vi "TDC读取_32b.vi"() -> ()   [LabVIEW 2014]
uses:
  <vilib>/Utility/file.llb/Write To Spreadsheet File (I64).vi
panel:
  in  "设定测量时间/秒":dbl
  out "测量进行时间/秒":dbl
  out "初始时间":u32
  in  "存储文件路径":path=path "C:/Users/Lebron/Desktop/tdc测试数据/Plain3/10ns.txt" caption="文件路径 （空时为对话框）"
  in  "停止":bool
  out "时间分布谱":dbl[](graph)
  in  "基路径":path=path "C:/Users/Lebron/Desktop/zxd/数据"
  out "路径":path
  in  "下拉列表":u16(ring) items=["继续", "停止"]
  out "状态":enum16{"空闲", "开始", "接收数据", "处理数据", "退出"}(ring)
  out "开关":bool
  in  "通道电压阈值":u16=500
  in  "开始":bool
  in  "初始状态":enum16{"空闲", "开始", "接收数据", "处理数据", "退出"}(ring)
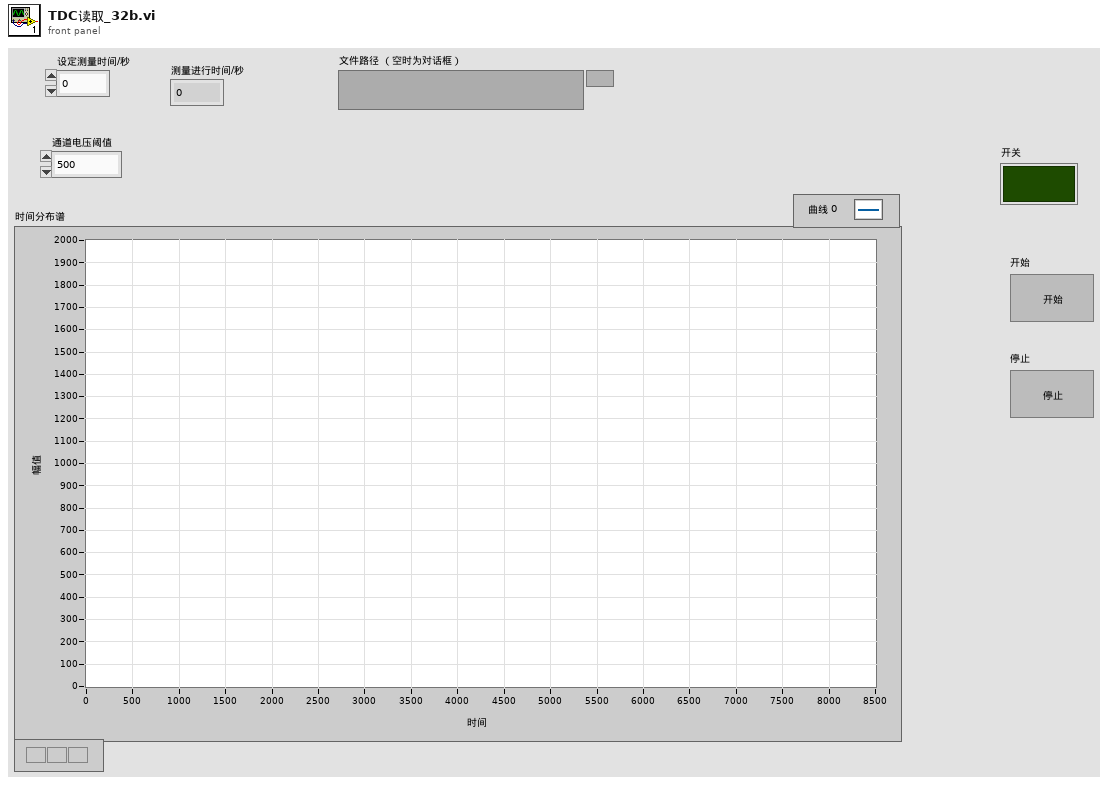
[diagram p1: front panel]
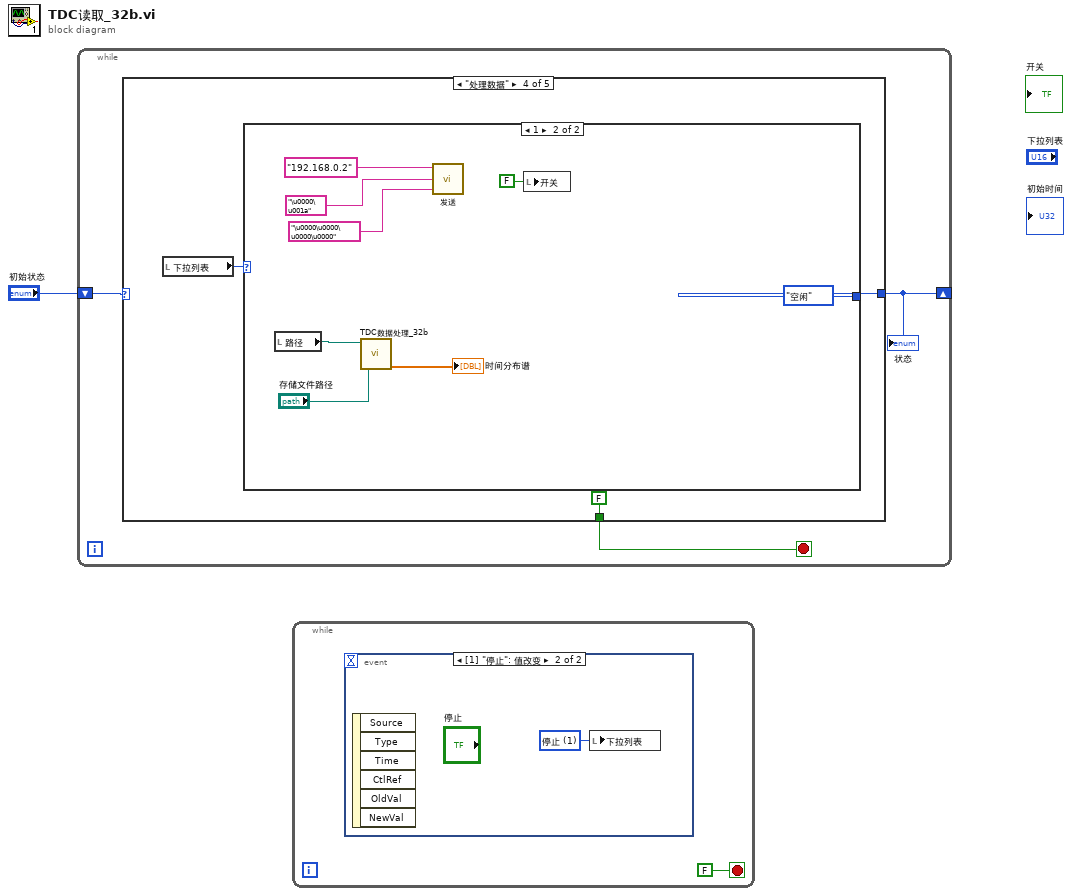
[diagram p0: block diagram]
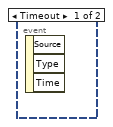
[diagram p2: hidden frame]
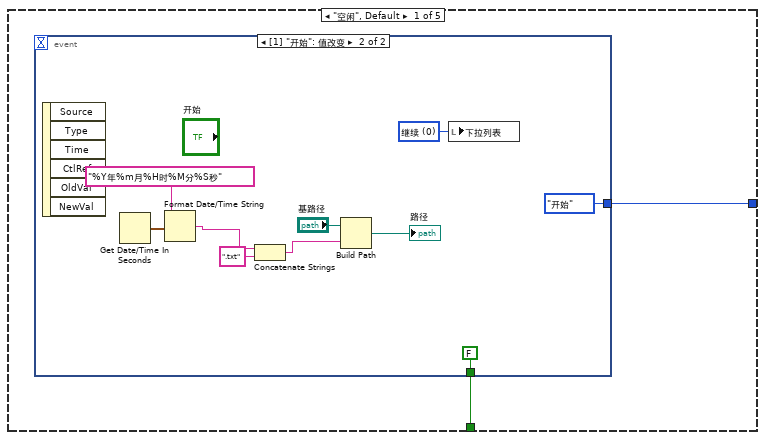
[diagram p3: hidden frame]
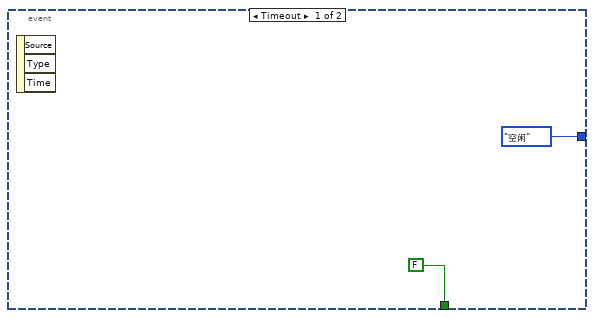
[diagram p4: hidden frame]
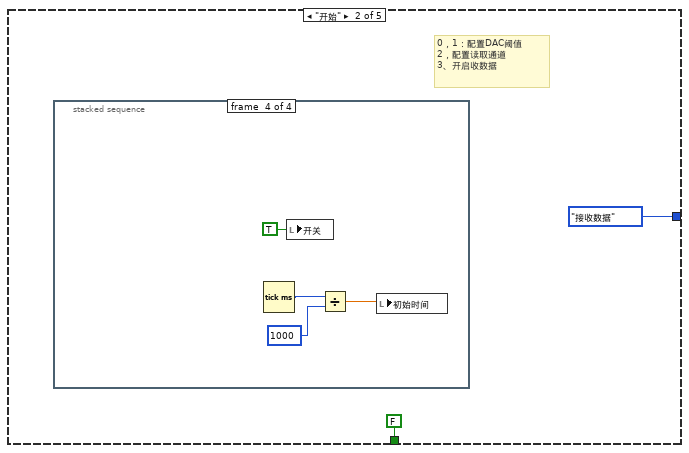
[diagram p5: hidden frame]
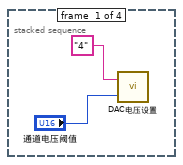
[diagram p6: hidden frame]
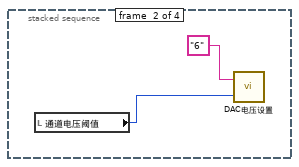
[diagram p7: hidden frame]
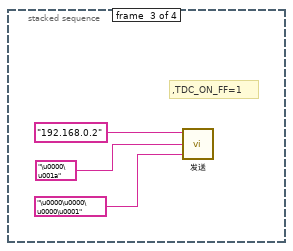
[diagram p8: hidden frame]
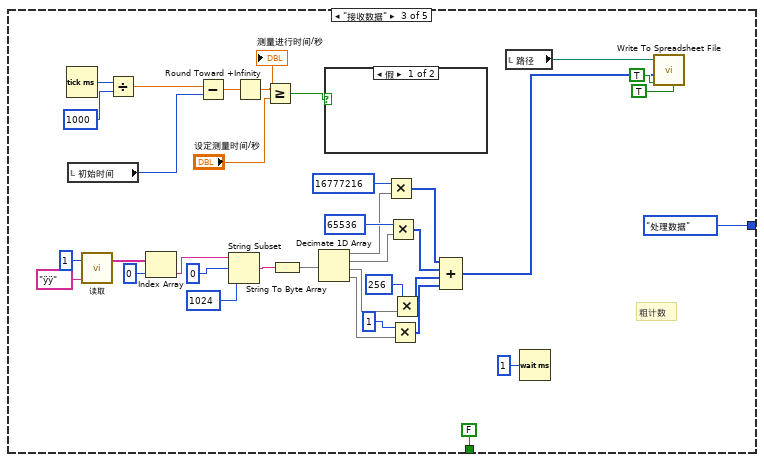
[diagram p9: hidden frame]
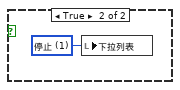
[diagram p10: hidden frame]
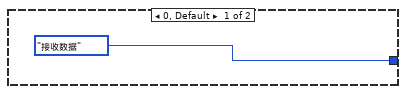
[diagram p11: hidden frame]
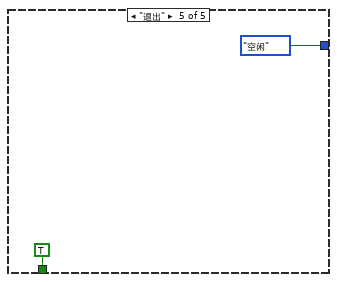
[diagram p12: hidden frame]
diagram:
  n1 = while {
    shift-right: [w3] -> _
    shift-left: "初始状态" -> [w4]
    stop <- w2 stop-if-true
    n2 = case shown="\"处理数据\"" w4 {
      tunnel: [w6 enum16{"空闲", "开始", "接收数据", "处理数据", "退出"}."接收数据" ("初始状态") enum16{"空闲", "开始", "接收数据", "处理数据", "退出"}."处理数据" ("初始状态") w70 enum16{"空闲", "开始", "接收数据", "处理数据", "退出"}."空闲" ("初始状态")] -> w3
      tunnel: [w5 FALSE FALSE FALSE TRUE] -> w2
      frame "空闲", Default {
        n3 = event shown="[1] \"开始\": 值改变" {
          selector: _ -> [_ _]
          dyn-events: _ -> [_ _]
          timeout: _ -> [_ _]
          tunnel: [enum16{"空闲", "开始", "接收数据", "处理数据", "退出"}."空闲" ("初始状态") enum16{"空闲", "开始", "接收数据", "处理数据", "退出"}."开始" ("初始状态")] -> w6
          tunnel: [FALSE FALSE] -> w5
          event Timeout {
            n4 = event-data() -> ()  [unwired: 1 in, 3 out]
          }
          event "开始": Value Change {
            w9 = u16 0 items=["继续", "停止"] ("下拉列表")
            n5 = event-data() -> ()  [unwired: 1 in, 6 out]
            n6 = Get Date/Time In Seconds() -> (seconds since 1Jan1904=w12:timestamp)
            n7 = Format Date/Time String(time format string (%c)="%Y年%m月%H时%M分%S秒" ("时间格式字符串(%c)"), seconds (now)=w12) -> (date/time string=w10:string)  [unwired: 1 in]
            n8 = Concatenate Strings(w10, ".txt" ("字符串")) -> (w14:string)
            n9 = Build Path(base path="基路径", name or relative path=w14) -> (appended path=→"路径":path)
            n10 = local write "下拉列表"(w9) -> ()
          }
        }
      }
      frame "开始" {
        # "0，1：配置DAC阈值\n2，配置读取通道\n3、开启收数据"
        n11 = stacked-sequence {
          frame #0 {
            n12 = call "DAC电压设置.vi"("电压"="通道电压阈值", "cmd_channel(8bit)"="4") -> ()  [unwired: 1 in]
          }
          frame #1 {
            n13 = local read "通道电压阈值"() -> (w23:u16)
            n14 = call "DAC电压设置.vi"("电压"=w23, "cmd_channel(8bit)"="6") -> ()  [unwired: 1 in]
          }
          frame #2 {
            # ",TDC_ON_FF=1"
            n15 = call "发送.vi"("数据（32bit）"="\u0000\u0000\u0000\u0001", "命令(16bit)"="\u0000\u001a", "目标IP"="192.168.0.2") -> ()  [unwired: 1 out]
          }
          frame #3 {
            n16 = Tick Count (ms)() -> (millisecond timer value=w30:u32)
            n17 = local write "开关"(TRUE ("开关")) -> ()
            n18 = Divide(x=w30, y=u32 1000) -> (x/y=w28:dbl)
            n19 = local write "初始时间"(w28) -> ()
          }
        }
      }
      frame "接收数据" {
        # "粗计数"
        n20 = Tick Count (ms)() -> (millisecond timer value=w39:u32)
        n21 = local read "初始时间"() -> (w36:u32)
        n22 = call "读取.vi"("命令"="ÿÿ", "帧数"=1) -> ("数组"=w66:string[])  [unwired: 1 out]
        n23 = Divide(x=w39, y=u32 1000) -> (x/y=w37:dbl)
        n24 = Index Array(array=w66, index=0 ("索引")) -> (element=w62:string)
        n25 = Subtract(x=w37, y=w36) -> (x-y=w35:dbl)
        n26 = String Subset(string=w62, offset (0)=0 ("偏移量(0)"), length (rest)=1024 ("长度（剩余）")) -> (substring=w61:string)
        n27 = Round Toward +Infinity(x=w35) -> (ceil(x): smallest int >= x=w34:dbl)
        "测量进行时间/秒" <- w34
        n28 = Greater Or Equal?(x=w34, y="设定测量时间/秒") -> (x >= y?=w33:bool)
        n29 = String To Byte Array(string=w61) -> (unsigned byte array=w60:u8[])
        n30 = Decimate 1D Array(w60) -> (w43:u8[], w44:u8[], w55:u8[], w54:u8[])
        n31 = case shown="假" w33 {
          frame False {
          }
          frame True {
            w68 = u16 1 items=["继续", "停止"] ("下拉列表")
            n32 = local write "下拉列表"(w68) -> ()
          }
        }
        n33 = Multiply(x=u32 16777216, y=w43) -> (x*y=w41:u32[])
        n34 = Multiply(x=u32 65536, y=w44) -> (x*y=w42:u32[])
        n35 = Multiply(x=u32 1, y=w54) -> (x*y=w52:u32[])
        n36 = Multiply(x=u32 256, y=w55) -> (x*y=w53:u32[])
        n37 = Compound Arithmetic op=ADD(w41, w42, w53, w52) -> (w47:u32[])
        n38 = local read "路径"() -> (w49:path)
        n39 = Wait (ms)(milliseconds to wait=u32 1 ("等待时间（毫秒）")) -> ()  [unwired: 1 out]
        n40 = call-poly <vilib>:"Write To Spreadsheet File.vi"("transpose? (no:F)"=TRUE, "append to file? (new file:F)"=TRUE, "1D data"=w47, "file path (dialog if empty)"=w49) -> ()  [unwired: 4 in, 1 out]
      }
      frame "处理数据" {
        n41 = local read "下拉列表"() -> (w69:u16)
        n42 = case shown="1" w69 {
          tunnel: [enum16{"空闲", "开始", "接收数据", "处理数据", "退出"}."接收数据" ("初始状态") enum16{"空闲", "开始", "接收数据", "处理数据", "退出"}."空闲" ("初始状态")] -> w70
          frame 0, Default {
          }
          frame 1 {
            n43 = local read "路径"() -> (w75:path)
            n44 = call "TDC数据处理_32b.vi"("存储文件路径"="存储文件路径", "路径"=w75) -> ("时间分布谱"=→"时间分布谱":dbl[])  [unwired: 3 in, 2 out]
            n45 = call "发送.vi"("数据（32bit）"="\u0000\u0000\u0000\u0000", "命令(16bit)"="\u0000\u001a", "目标IP"="192.168.0.2") -> ()  [unwired: 1 out]
            n46 = local write "开关"(FALSE ("开关")) -> ()
          }
        }
      }
      frame "退出" {
      }
    }
    "状态" <- w3
  }
  n47 = while {
    stop <- FALSE stop-if-true
    n48 = event shown="[1] \"停止\": 值改变" {
      selector: _ -> [_ _]
      dyn-events: _ -> [_ _]
      timeout: _ -> [_ _]
      event Timeout {
        n49 = event-data() -> ()  [unwired: 1 in, 3 out]
      }
      event "停止": Value Change {
        w84 = u16 1 items=["继续", "停止"] ("下拉列表")
        n50 = event-data() -> ()  [unwired: 1 in, 6 out]
        n51 = local write "下拉列表"(w84) -> ()
      }
    }
  }
